vi "getConfig.vi"() -> (0 "config":T1)   [LabVIEW 2015]
uses:
  <vilib>/Utility/config.llb/Read Key (String).vi
  <vilib>/Utility/config.llb/Read Key (I32).vi
  <vilib>/Utility/config.llb/NI_LVConfig.lvlib
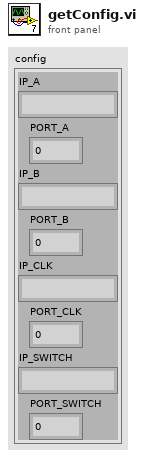
[diagram p1: front panel]
types:
  T1 = cluster{"IP_A":string, "PORT_A":i32, "IP_B":string, "PORT_B":i32, "IP_CLK":string, "PORT_CLK":i32, "IP_SWITCH":string, "PORT_SWITCH":i32}
  T2 = enum32{"invalid app kind", "Development System", "Run Time System", "Student Edition", "Embedded LabVIEW", "Evaluation", "Custom"}
  T3 = typedef "NI_LVConfig.lvlib/Config Data RefNum.ctl" = refnum<k1>
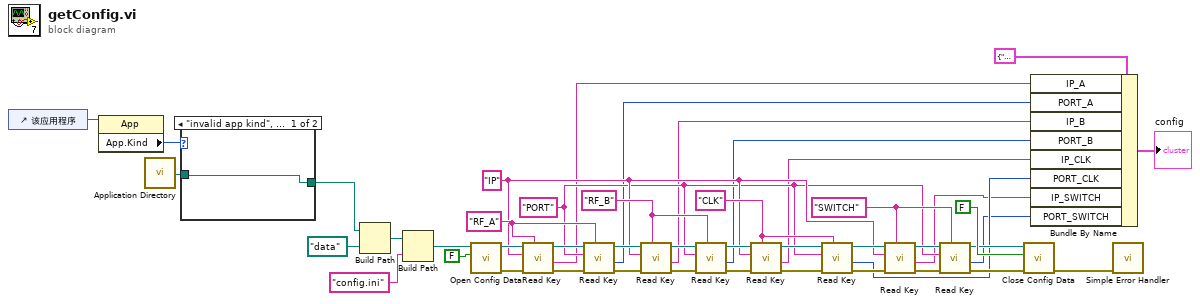
[diagram p0: block diagram]
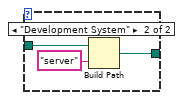
[diagram p2: hidden frame]
diagram:
  w24 = "SWITCH" ("section")
  w31 = "CLK" ("section")
  w20 = "PORT" ("键1")
  w32 = "RF_B" ("section")
  w35 = "RF_A" ("section")
  w21 = "IP" ("键1")
  n1 = control-ref of="该应用程序"() -> (w5:refnum<vi>)
  n2 = property class="App"(reference=w5) -> ("App.Kind"=w4:T2)  [unwired: 1 in, 2 out]
  n3 = call <vilib>:"Application Directory.vi"() -> ("Application Directory"=w3:path)
  n4 = case shown="\"invalid app kind\", 默认" w4 {
    tunnel: [w46 w47] -> w2
    tunnel: w3 -> [w46 w49]
    frame "invalid app kind", Default {
    }
    frame "Development System" {
      n5 = Build Path(base path=w49, name or relative path="server" ("名称或相对路径")) -> (appended path=w47:path)
    }
  }
  n6 = Build Path(base path=w2, name or relative path=path "data" ("default name")) -> (appended path=w41:path)
  n7 = Build Path(base path=w41, name or relative path="config.ini" ("名称或相对路径")) -> (appended path=w1:path)
  n8 = call <vilib>:"Open Config Data.vi"("create file if necessary (T)"=FALSE ("create file if necessary? (T)"), "configuration file path"=w1) -> ("error out"=w42:errorcluster, "refnum"=w43:T3)  [unwired: 7 in, 1 out]
  n9 = call-poly <vilib>:"Read Key.vi"("section"=w35, "error in (no error)"=w42, "key"=w21, "refnum"=w43) -> ("error out"=w36:errorcluster, "value"=w14:string, "refnum out"=w37:T3)  [unwired: 2 in, 3 out]
  n10 = call-poly <vilib>:"Read Key.vi"("section"=w35, "error in (no error)"=w36, "key"=w20, "refnum"=w37) -> ("error out"=w33:errorcluster, "value"=w13:i32, "refnum out"=w34:T3)  [unwired: 1 in, 4 out]
  n11 = call-poly <vilib>:"Read Key.vi"("section"=w32, "error in (no error)"=w33, "key"=w21, "refnum"=w34) -> ("error out"=w38:errorcluster, "value"=w12:string, "refnum out"=w39:T3)  [unwired: 2 in, 3 out]
  n12 = call-poly <vilib>:"Read Key.vi"("section"=w32, "error in (no error)"=w38, "key"=w20, "refnum"=w39) -> ("error out"=w27:errorcluster, "value"=w11:i32, "refnum out"=w28:T3)  [unwired: 1 in, 4 out]
  n13 = call-poly <vilib>:"Read Key.vi"("section"=w31, "error in (no error)"=w27, "key"=w21, "refnum"=w28) -> ("error out"=w30:errorcluster, "value"=w10:string, "refnum out"=w29:T3)  [unwired: 2 in, 3 out]
  n14 = call-poly <vilib>:"Read Key.vi"("section"=w31, "error in (no error)"=w30, "key"=w20, "refnum"=w29) -> ("error out"=w22:errorcluster, "value"=w9:i32, "refnum out"=w23:T3)  [unwired: 1 in, 4 out]
  n15 = call-poly <vilib>:"Read Key.vi"("section"=w24, "error in (no error)"=w22, "key"=w21, "refnum"=w23) -> ("error out"=w25:errorcluster, "value"=w8:string, "refnum out"=w26:T3)  [unwired: 2 in, 3 out]
  n16 = call-poly <vilib>:"Read Key.vi"("section"=w24, "error in (no error)"=w25, "key"=w20, "refnum"=w26) -> ("error out"=w17:errorcluster, "value"=w7:i32, "refnum out"=w16:T3)  [unwired: 1 in, 4 out]
  n17 = call <vilib>:"Close Config Data.vi"("error in (no error)"=w17, "write file if changed (T)"=FALSE ("write configuration file? (T)"), "refnum"=w16) -> ("error out"=w19:errorcluster)  [unwired: 8 out]
  n18 = Bundle By Name(cluster=T1 {"IP_A"="192.168.1.200", "PORT_A"=5000, "IP_B"="192.168.1.202", "PORT_B"=5000, "IP_CLK"="192.168.1.201", "PORT_CLK"=5000, "IP_SWITCH"="192.168.1.203", "PORT_SWITCH"=5000} ("config"), "IP_A"=w14, "PORT_A"=w13, "IP_B"=w12, "PORT_B"=w11, "IP_CLK"=w10, "PORT_CLK"=w9, "IP_SWITCH"=w8, "PORT_SWITCH"=w7) -> (→"config":T1)
  n19 = call <vilib>:"Simple Error Handler.vi"("error in (no error)"=w19) -> ()  [unwired: 1 in, 8 out]
